vi "VisualInspectionAHUold.vi"(8 "error in (no error)":errorcluster, 11 "TableRef":refnum<vi>) -> (0 "error out":errorcluster, 2 "VisualInspectionResult":bool)   [LabVIEW 2017]
panel:
  in  "Cancel Button":bool
  in  "OK Button":bool
  in  "7.5.1.1":bool
  in  "7.3":bool
  in  "7.2.3":bool
  in  "7.2.4":bool
  in  "7.2.5":bool
  in  "6.2.2.1":bool
  in  "6.2.2.2":bool
  in  "6.2.2.3":bool
  in  "6.2.2.4":bool
  in  "7.1":bool
  in  "6.2.1.1":bool
  in  "7.2.2":bool
  in  "6.1.2":bool
  in  "7.2.1.1":bool
  in  "7.2.1":bool
  in  "6.1.1":bool
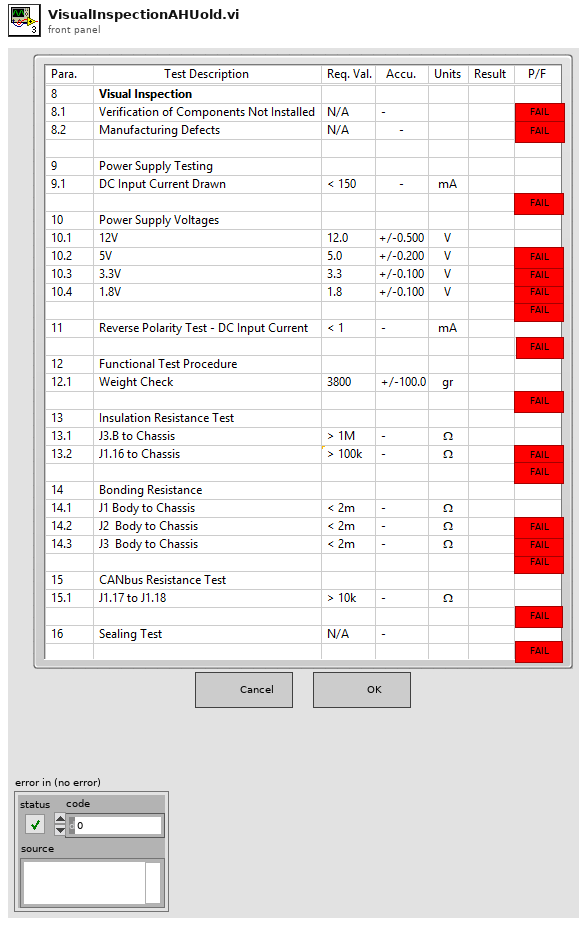
[diagram p1: front panel]
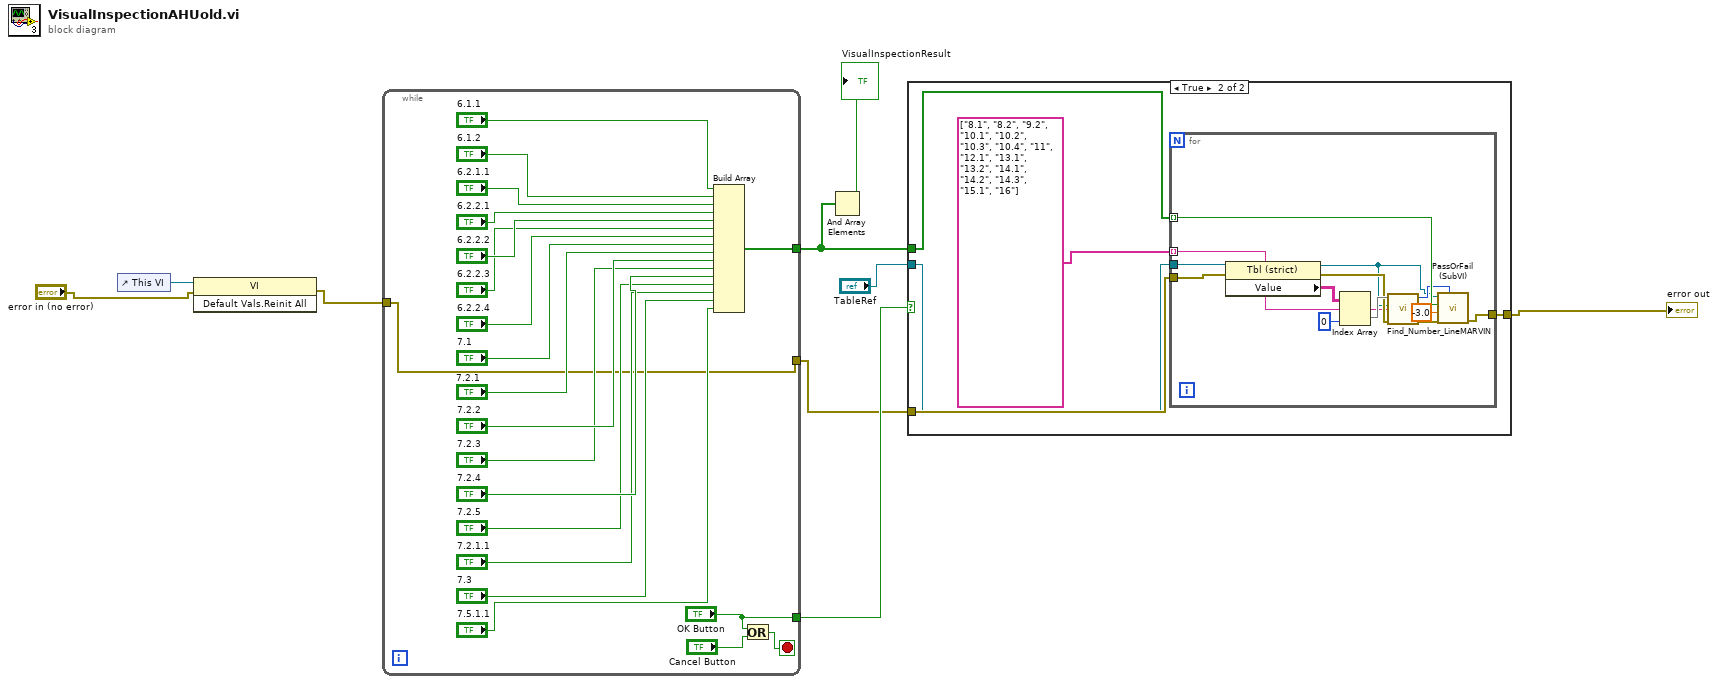
[diagram p0: block diagram]
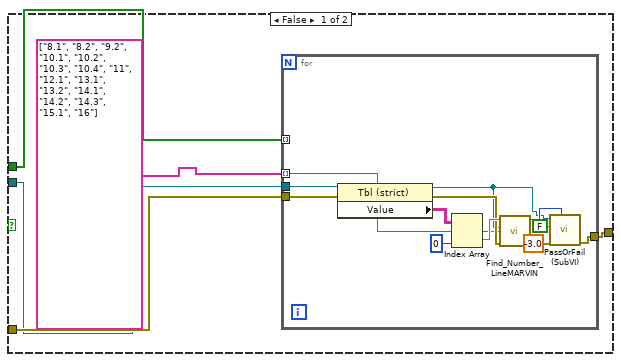
[diagram p2: hidden frame]
diagram:
  n1 = control-ref of="This VI"() -> (w5:refnum<vi>)
  n2 = invoke class="VI" method="Default Vals.Reinit All"(reference=w5, error in="error in (no error)") -> (error out=w9:errorcluster)  [unwired: 1 in, 2 out]
  n3 = while {
    tunnel: w9 -> [w10]
    tunnel: [w12] -> w2
    tunnel: ["OK Button"] -> w8
    tunnel: [w10] -> w7
    stop <- w29 stop-if-true
    n4 = Build Array("6.1.1", "6.1.2", "6.2.1.1", "6.2.2.1", "6.2.2.2", "6.2.2.3", "6.2.2.4", "7.1", "7.2.1", "7.2.2", "7.2.3", "7.2.4", "7.2.5", "7.2.1.1", "7.3", "7.5.1.1") -> (w12:bool[])
    n5 = Or(x="OK Button", y="Cancel Button") -> (x .or. y?=w29:bool)
  }
  n6 = And Array Elements(Boolean array=w2) -> (logical AND=→"VisualInspectionResult":bool)
  n7 = case shown="True" w8 {
    tunnel: w2 -> [w35 w53]
    tunnel: w7 -> [w34 w52]
    tunnel: [w33 w51] -> w3
    tunnel: "TableRef" -> [w32 w50]
    frame False {
      n8 = for {
        tunnel: string[] ["8.1", "8.2", "9.2", "10.1", "10.2", "10.3", "10.4", "11", "12.1", "13.1", "13.2", "14.1", "14.2", "14.3", "15.1", "16"] ("Array 3") -> [w44] mode=indexing
        tunnel: w35 -> [_] mode=indexing
        tunnel: w34 -> [w41]
        tunnel: [w40] -> w33
        tunnel: w32 -> [w39]
        n9 = property class="Tbl (strict)"(reference=w39, error in=w41) -> (reference out=w36:refnum<vi>, error out=w45:errorcluster, "Value"=w48:string[][])
        n10 = Index Array(array=w48, index (col)=0 ("disabled index (col)")) -> (element=w46:string[])  [unwired: 1 in]
        n11 = call "Find_Number_LineMARVIN.vi"("Test Paragraph"=w44, "error in"=w45, "TableIn"=w36, "Row Headers[]"=w46) -> ("error out"=w43:errorcluster, "Line number"=w42:i32)  [unwired: 1 in, 2 out]
        n12 = call "PassOrFail (SubVI).vi"("index (row)"=w42, "error in (no error)"=w43, "Data in"=-3.0, "Pass?Fail"=FALSE ("Boolean"), "Table in"=w36) -> ("error out"=w40:errorcluster)  [unwired: 6 in]
      }
    }
    frame True {
      n13 = for {
        tunnel: string[] ["8.1", "8.2", "9.2", "10.1", "10.2", "10.3", "10.4", "11", "12.1", "13.1", "13.2", "14.1", "14.2", "14.3", "15.1", "16"] ("Array 3") -> [w62] mode=indexing
        tunnel: w53 -> [w60] mode=indexing
        tunnel: w52 -> [w58]
        tunnel: [w57] -> w51
        tunnel: w50 -> [w56]
        n14 = property class="Tbl (strict)"(reference=w56, error in=w58) -> (reference out=w54:refnum<vi>, error out=w63:errorcluster, "Value"=w66:string[][])
        n15 = Index Array(array=w66, index (col)=0 ("disabled index (col)")) -> (element=w64:string[])  [unwired: 1 in]
        n16 = call "Find_Number_LineMARVIN.vi"("Test Paragraph"=w62, "error in"=w63, "TableIn"=w54, "Row Headers[]"=w64) -> ("error out"=w61:errorcluster, "Line number"=w59:i32)  [unwired: 1 in, 2 out]
        n17 = call "PassOrFail (SubVI).vi"("index (row)"=w59, "error in (no error)"=w61, "Data in"=-3.0, "Pass?Fail"=w60, "Table in"=w54) -> ("error out"=w57:errorcluster)  [unwired: 6 in]
      }
    }
  }
  "error out" <- w3
